vi "niRFUtil ERR Ignore an Error.vi"(6 "pre-read error":errorcluster, 8 "post-read error":errorcluster, 11 "Error Code":T1) -> (0 "error out":errorcluster, 3 "Error Ignored":bool)   [LabVIEW 2015, in "niRFUtil.lvlib"]
doc: "This utility ignores an error, given the error code input.\n\n(c) Copyright 2006, National Instruments, Inc. This VI may not be duplicated, sold, or distributed without written consent from National Instruments."
uses:
  niRFUtil.lvlib
  Includes/niRFUtil INC Error Code.ctl
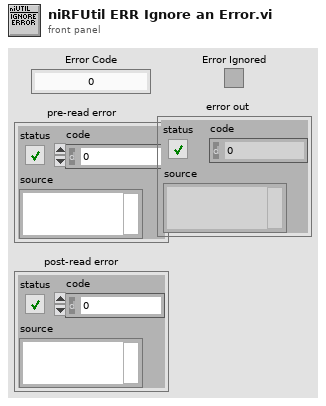
[diagram p1: front panel]
types:
  T1 = typedef "niRFUtil.lvlib/niRFUtil INC Error Code.ctl" = i32
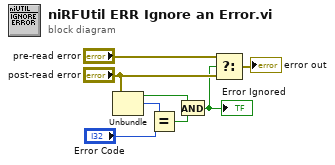
[diagram p0: block diagram]
diagram:
  n1 = Unbundle("post-read error") -> ("status"=w6:bool, "code"=w8:i32)  [unwired: 1 out]
  n2 = Equal?(x=w8, y="Error Code") -> (x = y?=w7:bool)
  n3 = And(x=w6, y=w7) -> (x .and. y?=w2:bool)
  "Error Ignored" <- w2
  n4 = Select(t="pre-read error", s=w2, f="post-read error") -> (s? t:f=→"error out":errorcluster)
